vi "Is Flat Type.vi"(8 "error in (no error)":errorcluster, 11 "LVEnum in":refnum<class "LVEnum.lvclass">) -> (0 "error out":errorcluster, 2 "Flat Type?":bool, 3 "LVEnum out":refnum<class "LVEnum.lvclass">)   [LabVIEW 2020, in "LVDataTypes.lvlib" / "LVEnum.lvclass"]
uses:
  <vilib>/AppBuilder/Engine/WebServiceDescription/LVDataTypes/LVEnum/LVEnum.lvclass
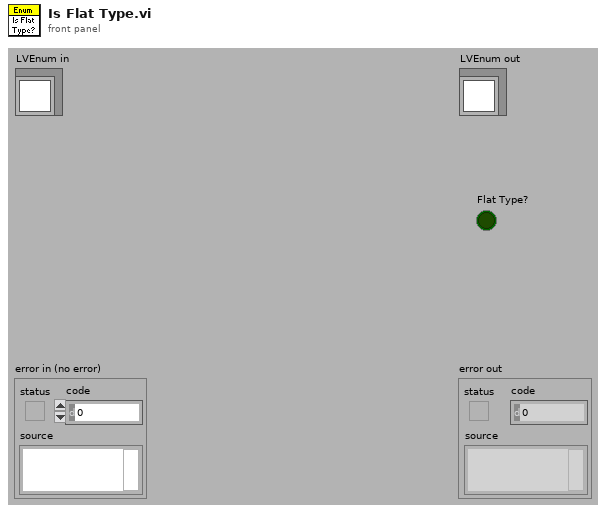
[diagram p1: front panel]
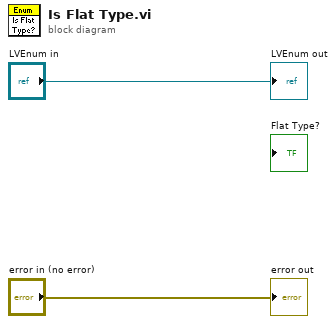
[diagram p0: block diagram]
diagram:
  "error out" <- "error in (no error)"
  "LVEnum out" <- "LVEnum in"
